vi "get Test by id.vi"(8 "error in (no error)":errorcluster caption="Fehler (Eingang, kein Fehler)", 10 "id":i32, 11 "Report (Eingang)":refnum<class "Report.lvclass">) -> (0 "error out":errorcluster caption="Fehler (Ausgang)", 1 "id found":bool, 2 "Test.lvclass":refnum<class "Test.lvclass">, 3 "Report (Ausgang)":refnum<class "Report.lvclass">, 4 "index":i32)   [LabVIEW 2013, in "DatenKlassen.lvlib" / "Report.lvclass"]
uses:
  Report.lvclass
  Test/Test.lvclass
  Report.lvclass/Report.ctl
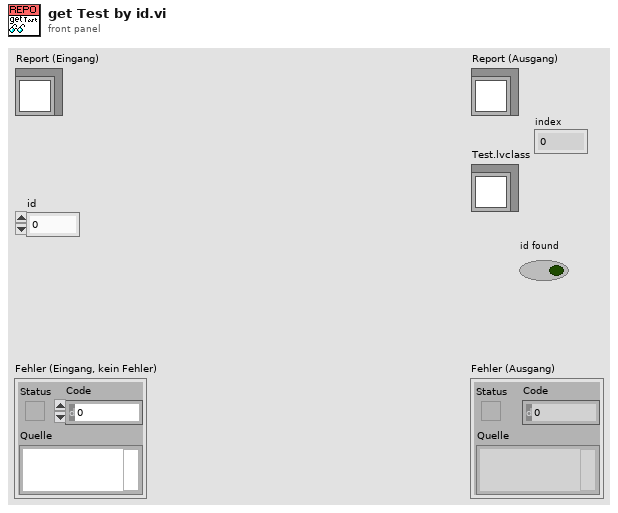
[diagram p1: front panel]
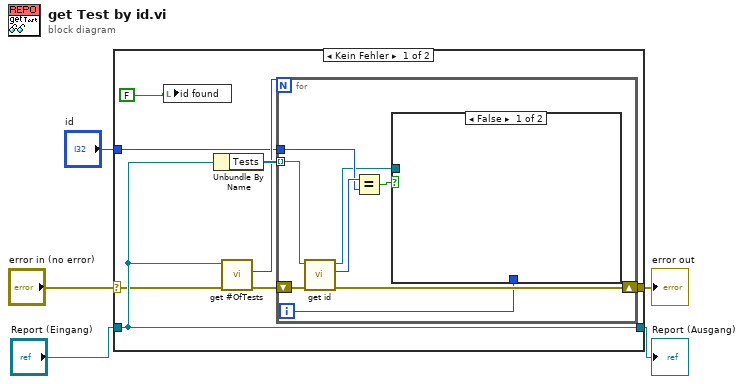
[diagram p0: block diagram]
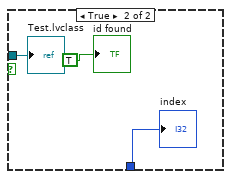
[diagram p2: hidden frame]
diagram:
  n1 = case shown="Kein Fehler" "error in (no error)" {
    selector: "error in (no error)" -> [w10 w25]
    tunnel: [w8 w25] -> w4
    tunnel: [w12 w26] -> w2
    tunnel: "Report (Eingang)" -> [w12 w26]
    tunnel: "id" -> [w7 _]
    frame No Error {
      n2 = local write "id found"(FALSE ("id found")) -> ()
      n3 = Unbundle By Name(w12) -> ("Tests"=w13:refnum<class "Test.lvclass">[])
      n4 = call-dynamic "get #OfTests.vi"("error in (no error)"=w10, "Report (Eingang)"=w12) -> ("error out"=w9:errorcluster, "#OfTests"=w11:u32)  [unwired: 7 in, 1 out]
      n5 = for {
        N: w11 -> [_]
        tunnel: w13 -> [w21] mode=indexing
        shift-right: [w19] -> w8
        shift-left: w9 -> [w20]
        tunnel: w7 -> [w17]
        i -> [w14]
        n6 = call-dynamic "get id.vi"("error in (no error)"=w20, "Test (Eingang)"=w21) -> ("error out"=w19:errorcluster, "id"=w18:i32, "Test (Ausgang)"=w15:refnum<class "Test.lvclass">)  [unwired: 7 in]
        n7 = Equal?(x=w18, y=w17) -> (x = y?=w16:bool)
        n8 = case shown="False" w16 {
          tunnel: w15 -> [_ w24]
          tunnel: w14 -> [_ w22]
          frame False {
          }
          frame True {
            "Test.lvclass" <- w24
            "id found" <- TRUE
            "index" <- w22
          }
        }
      }
    }
    frame Error {
    }
  }
  "error out" <- w4
  "Report (Ausgang)" <- w2
